vi "Set Dynamic Parameters.vi"(8 "error in (no error)":errorcluster, 10 "dynamic parameters":T2={"mass"=0.0, "gear ratio"=0.0, "motor inertia"=0.0, "center of gravity"=[], "viscous friction"=0.0, "positive coulomb friction"=0.0, "negative coulomb friction"=0.0, "inertia matrix"=[[0.0, 0.0, 0.0], [0.0, 0.0, 0.0], [0.0, 0.0, 0.0]]}, 11 "link in":refnum<class "NI_Robotics_Link.lvclass">) -> (0 "error out":errorcluster, 3 "link out":refnum<class "NI_Robotics_Link.lvclass">)   [LabVIEW 2017, in "NI_Robotics_Link.lvclass"]
doc: "<B>Use the Initialize Serial Arm VI instead of this VI to create and modify serial arms.</B>\n\nDefines the dynamic properties of a robotic arm link and the joint at the end of the link. To perform dynamic calculations for a robotic arm, you must specify the dynamic properties of each link and joint pair.\n\n<B>.m file:</B> link\n\n<B>link in</B> is a reference to a serial robotic arm link. \n<B>dynamic parameters</B> is a cluster whose elements define the dynamic properties of the link. \n <B>mass</B> specifies the mass of the link. \n <B>gear ratio</B> specifies the ratio of motor velocity to joint velocity. \n <B>motor inertia</B> specifies the force required to accelerate or decelerate the motor. \n <B>center of gravity</B> is a three-element array that defines the point on the link at which the weight of the link can be considered to act. \n <B>viscous friction</B> specifies the force of resistance of joint surfaces in motion through a fluid. \n <B>positive coulomb friction</B> specifies the force of resistance between dry joint surfaces in the positive direction. \n <B>negative coulomb friction</B> specifies the force of resistance between dry joint surfaces in the negative direction. \n <B>inertia matrix</B> specifies the torque that results from inertia on the link. \n<B>error in</B> describes error conditions that occur before this node runs. This input provides standard error in functionality. \n<B>link out</B> is a reference to a serial robotic arm link. You can wire this output to other Serial Arm Definition VIs. \n<B>error out</B> contains error information. This output provides standard error out functionality."
uses:
  <vilib>/robotics/Kinematics/Link/NI_Robotics_Link.lvclass
  <vilib>/Analysis/Matrix/Datatypes/RealMatrix.ctl
  <vilib>/robotics/Kinematics/Link/NI_Robotics_Link.lvclass/NI_Robotics_Link.ctl
  <vilib>/robotics/Utilities/NI_Robotics Utilities.lvlib
  <vilib>/Analysis/Matrix/NI_Matrix.lvlib
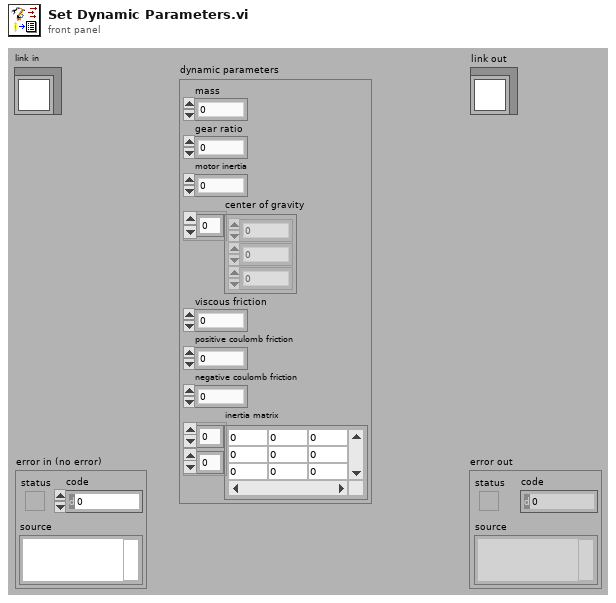
[diagram p1: front panel]
types:
  T1 = typedef "NI_Matrix.lvlib/RealMatrix.ctl" = dbl[][]
  T2 = cluster{"mass":dbl, "gear ratio":dbl, "motor inertia":dbl, "center of gravity":dbl[], "viscous friction":dbl, "positive coulomb friction":dbl, "negative coulomb friction":dbl, "inertia matrix":T1}
  T3 = cluster{"positive coulomb friction":dbl, "negative coulomb friction":dbl}
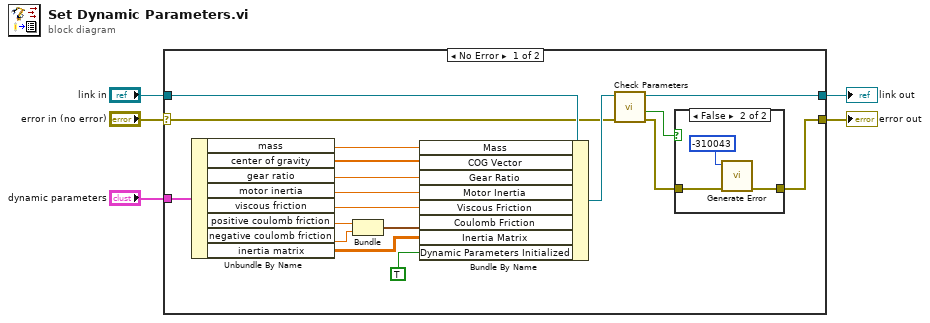
[diagram p0: block diagram]
diagram:
  n1 = case shown="No Error" "error in (no error)" {
    selector: "error in (no error)" -> [w8 w28]
    tunnel: [w13 w28] -> w4
    tunnel: [w9 w29] -> w2
    tunnel: "link in" -> [w23 w29]
    tunnel: "dynamic parameters" -> [w19 _]
    frame No Error {
      n2 = Unbundle By Name(w19) -> ("mass"=w17:dbl, "center of gravity"=w18:dbl[], "gear ratio"=w22:dbl, "motor inertia"=w21:dbl, "viscous friction"=w16:dbl, "positive coulomb friction"=w15:dbl, "negative coulomb friction"=w14:dbl, "inertia matrix"=w12:T1)
      n3 = Bundle("positive coulomb friction"=w15, "negative coulomb friction"=w14) -> (w20:T3)  [unwired: 1 in]
      n4 = Bundle By Name(cluster=w23, "Mass"=w17, "COG Vector"=w18, "Gear Ratio"=w22, "Motor Inertia"=w21, "Viscous Friction"=w16, "Coulomb Friction"=w20, "Inertia Matrix"=w12, "Dynamic Parameters Initialized"=TRUE) -> (w10:refnum<class "NI_Robotics_Link.lvclass">)
      n5 = call-dynamic "Check Parameters.vi"("error in (no error)"=w8, "link in"=w10) -> ("error out"=w7:errorcluster, "dynamics valid"=w6:bool, "lin out"=w9:refnum<class "NI_Robotics_Link.lvclass">)  [unwired: 6 in, 1 out]
      n6 = case shown="False" w6 {
        tunnel: w7 -> [w24 w27]
        tunnel: [w24 w26] -> w13
        frame True {
        }
        frame False {
          n7 = call <vilib>:"Generate Error.vi"("error in (no error)"=w27, "code"=-310043) -> ("error out"=w26:errorcluster)  [unwired: 9 in]
        }
      }
    }
    frame Error {
    }
  }
  "error out" <- w4
  "link out" <- w2
